vi "ConnectToServer.vi"(6 "client key":string="dGhlIHNhbXBsZSBub25jZQ==", 8 "error in":errorcluster, 10 "port":u16=9090, 11 "address":string="192.168.1.7") -> (0 "error out":errorcluster, 2 "status line":string, 3 "connection ID":refnum<k5>, 5 "header":string)   [LabVIEW 2014, in "Raspberry Pi Compatible Compiler for LabVIEW.lvlib" / "Websocket.lvlib"]
uses:
  Websocket.lvlib
panel:
  out "server key":string
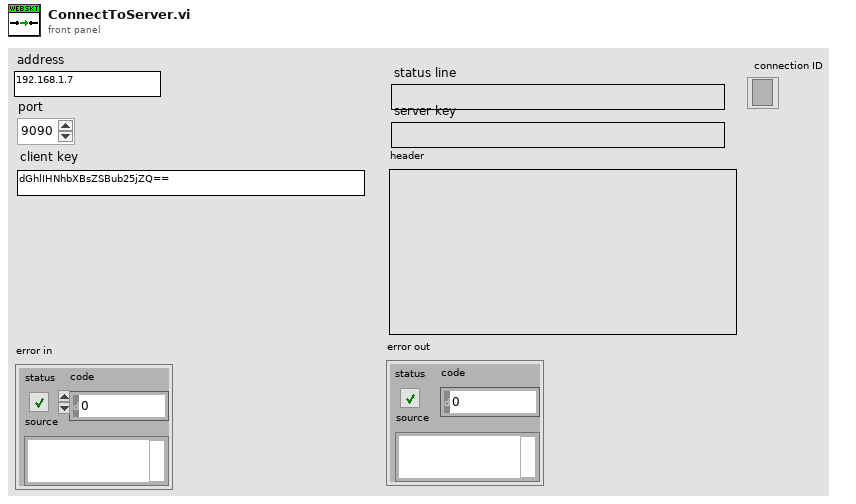
[diagram p1: front panel]
types:
  T1 = enum16{"Standard", "Buffered", "CRLF", "Immediate"}
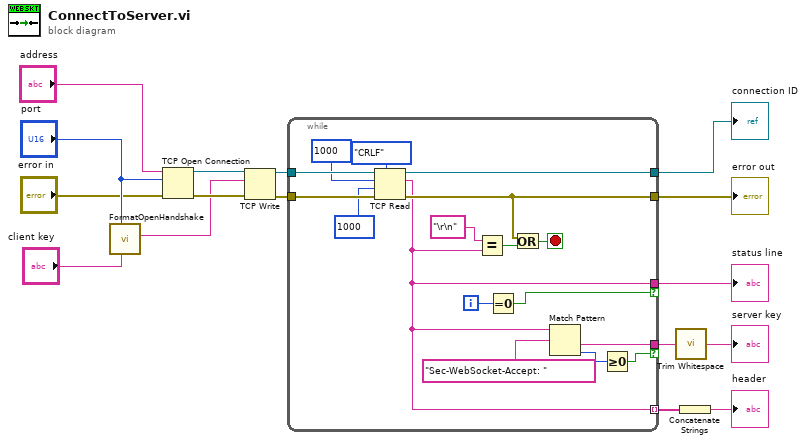
[diagram p0: block diagram]
diagram:
  n1 = call "FormatOpenHandshake.vi"("Websocket Key"="client key", "Port (9090)"="port") -> ("opening handshake"=w8:string)  [unwired: 9 in]
  n2 = TCP Open Connection(address="address", remote port or service name="port", error in (no error)="error in") -> (connection ID=w10:refnum<k5>, error out=w11:errorcluster)  [unwired: 2 in]
  n3 = TCP Write(connection ID=w10, data in=w8, error in (no error)=w11) -> (connection ID out=w12:refnum<k5>, error out=w13:errorcluster)  [unwired: 1 in, 1 out]
  n4 = while {
    tunnel: w12 -> [w33]
    tunnel: w13 -> [w32]
    tunnel: [w31] -> w3
    tunnel: [w26] -> w2
    tunnel: [w17] -> w14 mode=indexing
    tunnel: [w17] -> w7 if=w22
    tunnel: [w20] -> w6 if=w18
    i -> [w23]
    stop <- w24 stop-if-true
    n5 = TCP Read(connection ID=w33, bytes to read=1000, error in (no error)=w32, 7:T1."CRLF" ("mode (standard)"), 9:1000 ("timeout ms (25000)")) -> (connection ID out=w31:refnum<k5>, data out=w17:string, error out=w26:errorcluster)
    n6 = Equal?(x="\r\n", y=w17) -> (x = y?=w25:bool)
    n7 = Equal To 0?(x=w23) -> (x = 0?=w22:bool)
    n8 = Or(x=w26, y=w25) -> (x .or. y?=w24:bool)
    n9 = Match Pattern(string=w17, regular expression="Sec-WebSocket-Accept: ") -> (after substring=w20:string, offset past match=w19:i32)  [unwired: 1 in, 2 out]
    n10 = Greater Or Equal To 0?(x=w19) -> (x >= 0?=w18:bool)
  }
  "status line" <- w7
  "connection ID" <- w3
  "error out" <- w2
  n11 = call <vilib>:"Trim Whitespace.vi"("string"=w6) -> ("trimmed string"=→"server key":string)  [unwired: 1 in]
  n12 = Concatenate Strings(w14) -> (→"header":string)
